vi "BLE_ExtractData.vi"(0 "ServicesUUIDs Value":string[][](array[string]), 11 "error in (no error)":errorcluster) -> (4 "ServicesUUIDs Extract Value":string[][](table), 15 "error out":errorcluster)   [LabVIEW 2020, in "BLE.lvlib"]
uses:
  BLE.lvlib
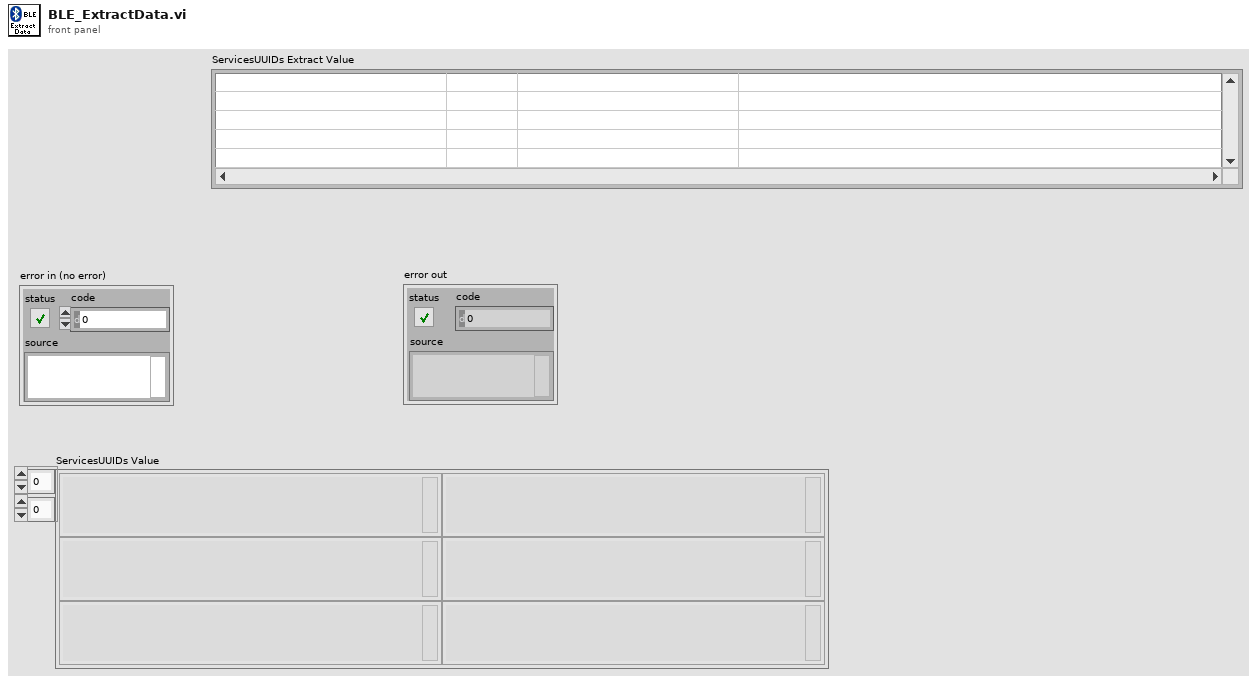
[diagram p1: front panel]
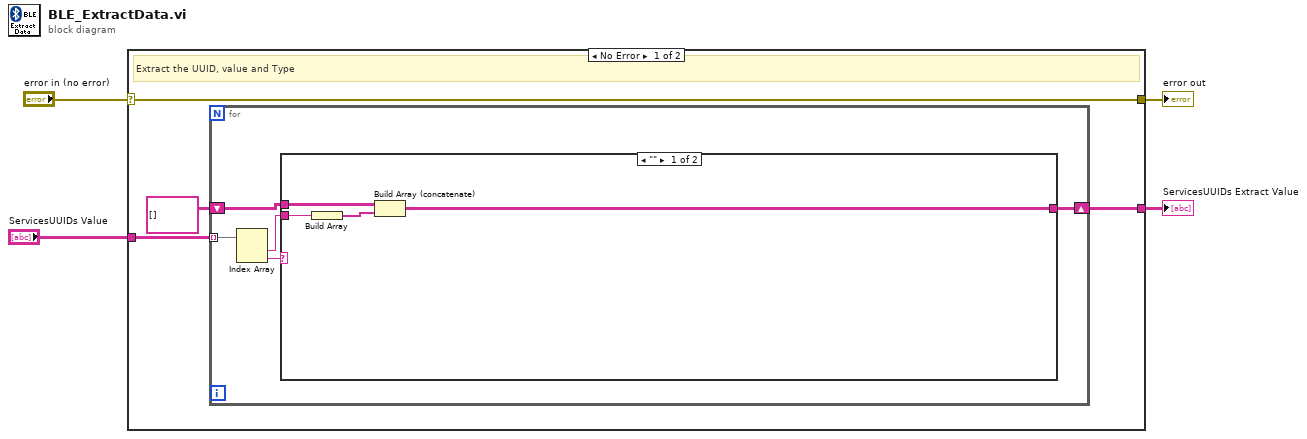
[diagram p0: block diagram]
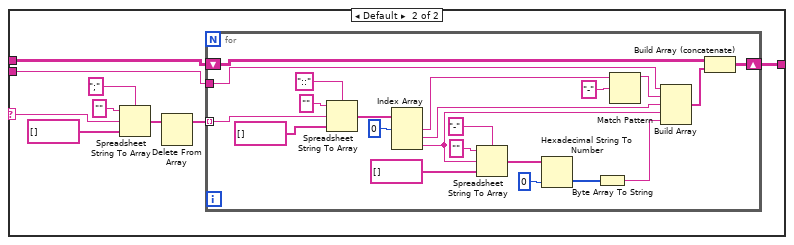
[diagram p2: hidden frame]
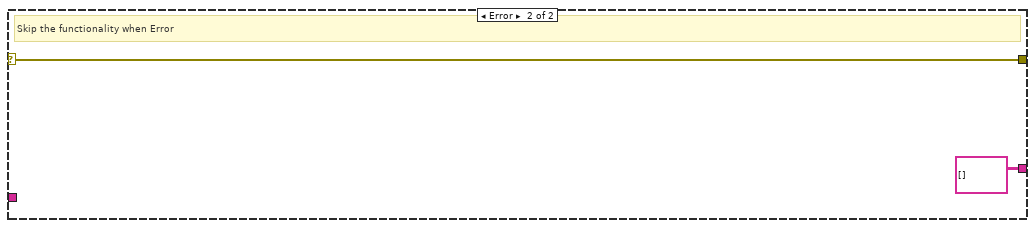
[diagram p3: hidden frame]
diagram:
  n1 = case shown="No Error" "error in (no error)" {
    selector: "error in (no error)" -> [w5 w50]
    tunnel: "ServicesUUIDs Value" -> [w8 _]
    tunnel: [w6 string[][] []] -> w3
    tunnel: [w5 w50] -> w2
    frame No Error {
      # "Extract the UUID, value and Type"
      n2 = for {
        tunnel: w8 -> [w13] mode=indexing
        shift-right: [w9] -> w6
        shift-left: string[][] [] -> [w10]
        n3 = Index Array(array=w13) -> (element #1=w11:string, element #2=w12:string)  [unwired: 2 in]
        n4 = case shown="\"\"" w12 {
          selector: w12 -> [_ w26]
          tunnel: w11 -> [w16 w22]
          tunnel: w10 -> [w15 w21]
          tunnel: [w14 w20] -> w9
          frame "" {
            n5 = Build Array(w16) -> (w17:string[])
            n6 = Build Array (concatenate)(w15, w17) -> (w14:string[][])
          }
          frame Default {
            n7 = Spreadsheet String To Array(delimiter (Tab)=";", format string="", spreadsheet string=w26, array type (2D Dbl)=string[] []) -> (array=w19:string[])
            n8 = Delete From Array(array=w19) -> (array with subset deleted=w18:string[])  [unwired: 2 in, 1 out]
            n9 = for {
              tunnel: w18 -> [w47] mode=indexing
              tunnel: w22 -> [w41]
              shift-right: [w35] -> w20
              shift-left: w21 -> [w36]
              n10 = Spreadsheet String To Array(delimiter (Tab)="::", format string="", spreadsheet string=w47, array type (2D Dbl)=string[] []) -> (array=w44:string[])
              n11 = Index Array(array=w44, index #1=0 ("index")) -> (element #1=w43:string, element #2=w38:string, element #3=w32:string)  [unwired: 2 in]
              n12 = Spreadsheet String To Array(delimiter (Tab)="-", format string="", spreadsheet string=w32, array type (2D Dbl)=string[] []) -> (array=w30:string[])
              n13 = Hexadecimal String To Number(string=w30, default (0uL)=u8 0 ("default (0 U32)")) -> (number=w28:u8[])  [unwired: 1 in, 1 out]
              n14 = Byte Array To String(unsigned byte array=w28) -> (string=w27:string)
              n15 = Match Pattern(string=w43, regular expression="-") -> (before substring=w40:string)  [unwired: 1 in, 3 out]
              n16 = Build Array(w41, w40, w38, w32, w27) -> (w37:string[])
              n17 = Build Array (concatenate)(w36, w37) -> (w35:string[][])
            }
          }
        }
      }
    }
    frame Error {
      # "Skip the functionality when Error"
    }
  }
  "ServicesUUIDs Extract Value" <- w3
  "error out" <- w2
